vi "Fetch Project Documentation.vi"(8 "error in (no error)":errorcluster {"code" format="Error %.0f"}, 11 "Project in":refnum<vi>) -> (0 "error out":errorcluster {"code" format="Error %.0f"}, 2 "Project Doc out":refnum<class "Project Documentation.lvclass">, 3 "Project out":refnum<vi>)   [LabVIEW 2023, in "VIDoc Parsing.lvlib" / "Project Documentation.lvclass"]
doc: "Takes a Project Reference in and parses out all Project Documentation information needed for document generation."
uses:
  Project Documentation.lvclass
  Project Documentation.lvclass/Project Documentation.ctl
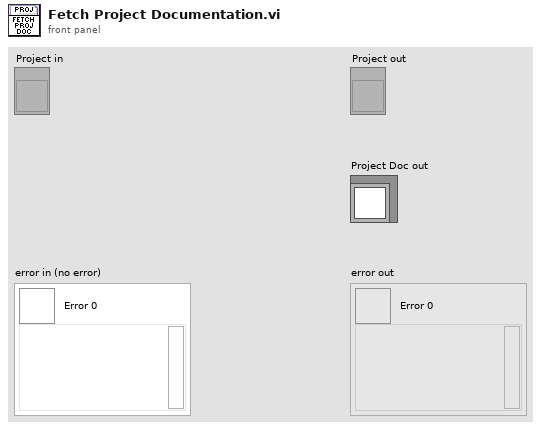
[diagram p1: front panel]
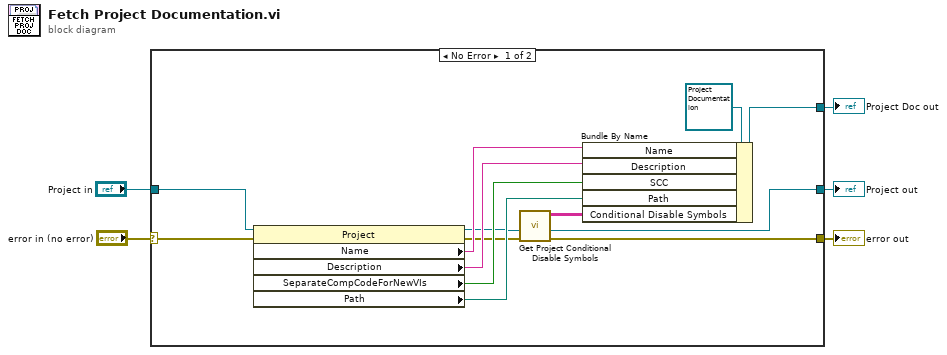
[diagram p0: block diagram]
diagram:
  n1 = case shown="No Error" "error in (no error)" {
    selector: "error in (no error)" -> [w6 w20]
    tunnel: [w16 w20] -> w4
    tunnel: "Project in" -> [w18 w19]
    tunnel: [w17 _] -> w2
    tunnel: [w15 w19] -> w1
    frame No Error {
      n2 = property class="Project"(reference=w18, error in=w6) -> (reference out=w9:refnum<vi>, error out=w8:errorcluster, "Name"=w13:string, "Description"=w12:string, "SeparateCompCodeForNewVIs"=w11:bool, "Path"=w10:path)
      n3 = call "Get Project Conditional Disable Symbols.vi"("error in (no error)"=w8, "Project in"=w9) -> ("error out"=w16:errorcluster, "Project out"=w15:refnum<vi>, "Conditional Disable Symbols"=w7:string[][])  [unwired: 7 in]
      n4 = Bundle By Name(cluster=refnum<class "Project Documentation.lvclass"> refnum ("Project Doc out"), "Name"=w13, "Description"=w12, "SCC"=w11, "Path"=w10, "Conditional Disable Symbols"=w7) -> (w17:refnum<class "Project Documentation.lvclass">)
    }
    frame Error {
    }
  }
  "error out" <- w4
  "Project Doc out" <- w2
  "Project out" <- w1
